vi "RemoteControl.TestLauncher.ConnectionMonitor.vi"(8 "error in (no error)":errorcluster, 11 "RC COM Type":T3=enum."ZMQ") -> (0 "error out":errorcluster)   [LabVIEW 2019, in "RemoteControl.lvclass"]
uses:
  RemoteControl.lvclass
  <vilib>/JKI/JKI SMO/SMO/Typedefs/SMOState --Enum.ctl
  Typedefs/PrivateEvents--RemoteControl.Configure.ctl
  Typedefs/RC Com Type--enum.ctl
  Typedefs/Message--Cluster.ctl
  Typedefs/RC Process Type--Enum.ctl
  RemoteControl.lvclass/RemoteControl.ctl
  <vilib>/JKI/JKI SMO/SMO/SMO.lvclass/SMO.ctl
  Typedefs/PrivateEvents--RemoteControl.SendMessageToProcess.ctl
  <vilib>/JKI/JKI SMO/SMO/Private/ReftoDVR--SMO.vi
  C:/Program Files (x86)/National Instruments/LabVIEW 2019/vi.lib/JKI/JKI SMO/SMO/SMO.lvclass
  <vilib>/JKI/JKI SMO/SMO/SMO.lvclass
panel:
  out "Response":T1={"Command"="Command3", "Data"=variant(string "Command: Command3\nTime: 10:01:32 AM\nGUID: 48148DED-56D8-49E7-9F94-E56068A2CC24"), "ID"="bc5bb9c457fa8484a73b80f0f0e9ae33"}
  in  "RC Process Type":T2=enum."Server"
  in  "Debug Mode":bool
  in  "Check Timing Mode":bool
  out "processed":i32=160
  out "Message":T1={"Command"="Command3", "Data"=variant(string[] ["[1433526]"]), "ID"="bc5bb9c457fa8484a73b80f0f0e9ae33"}
  in  "Configure":T4={"address"="*", "Port"=6341, "AllowedRemote"="", "Commands"=["Command1", "Command2", "Command3", "ACK", "HELP"], "timeout"=0}
  out "SMO State":T5=enum."Stopped"
  in  "Stop":bool
  # "RC SMO Test Launcher"
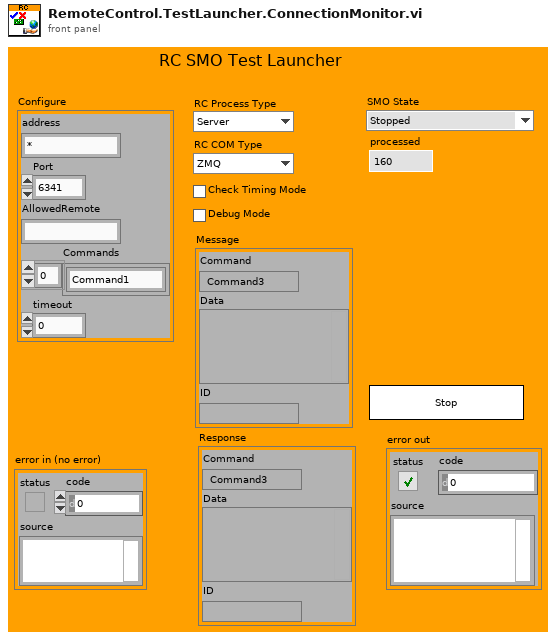
[diagram p1: front panel]
types:
  T1 = typedef "RemoteControl.lvclass/Message--Cluster.ctl" = cluster{"Command":string, "Data":variant, "ID":string}
  T2 = typedef "RemoteControl.lvclass/RC Process Type--Enum.ctl" = enum16{"Listener", "Server", "Client"}
  T3 = typedef "RemoteControl.lvclass/RC Com Type--enum.ctl" = enum16{"RC", "STM", "ZMQ"}
  T4 = typedef "RemoteControl.lvclass/PrivateEvents--RemoteControl.Configure.ctl" = cluster{"address":string, "Port":u16, "AllowedRemote":string, "Commands":string[], "timeout":i32}
  T5 = typedef "SMO.lvclass/SMOState --Enum.ctl" = enum16{"unknown", "Created", "Started", "Stopped"}
  T6 = typedef "SMO.lvclass/Public Events.ctl" = cluster{"Error":refnum<user-event>, "State":refnum<user-event>, "Reserve State":refnum<user-event>}
  T7 = typedef "RemoteControl.lvclass/PublicEvents--Cluster.ctl" = cluster{"SendMessageFromProcess":refnum<user-event>}
  T8 = typedef "RemoteControl.lvclass/PrivateEvents--RemoteControl.SendMessageToProcess.ctl" = cluster{"Message":T1}
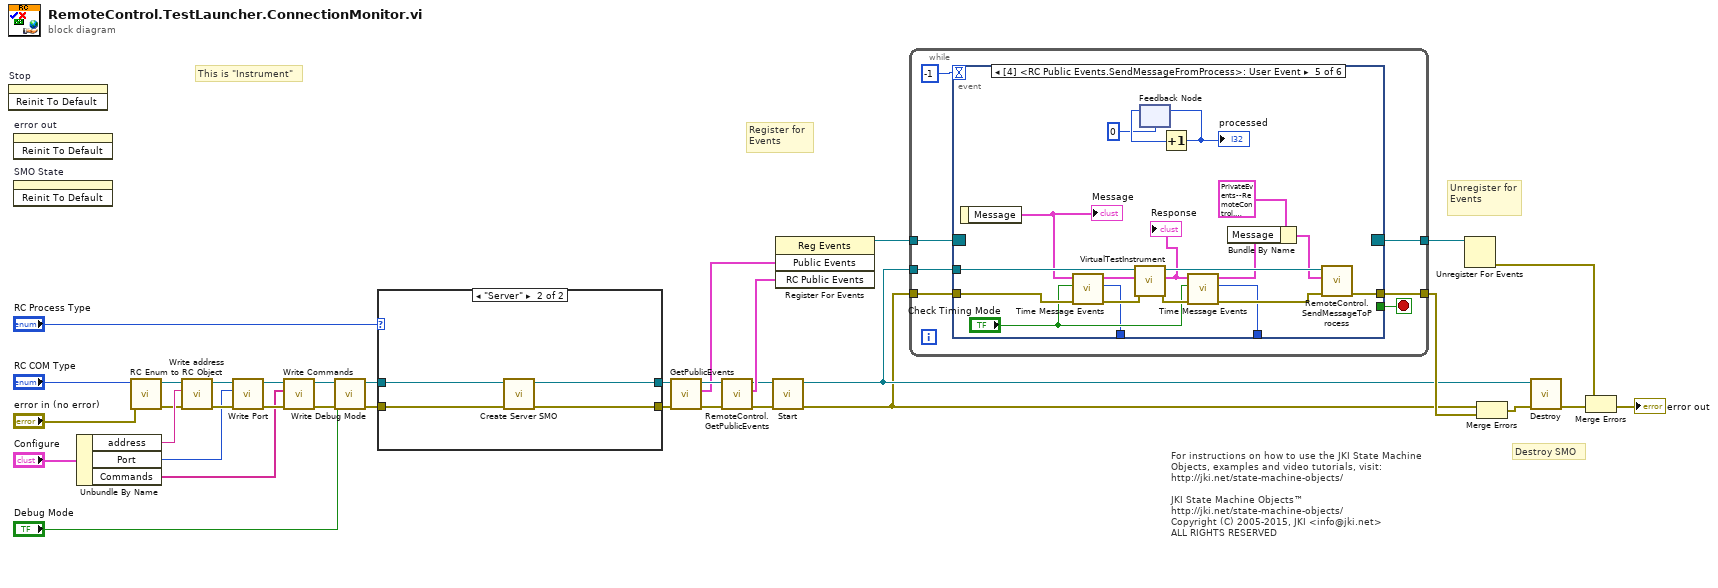
[diagram p0: block diagram]
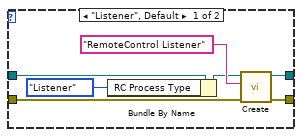
[diagram p2: hidden frame]
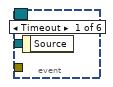
[diagram p3: hidden frame]
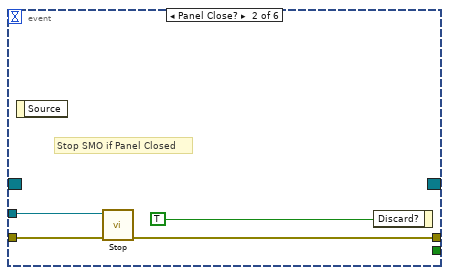
[diagram p4: hidden frame]
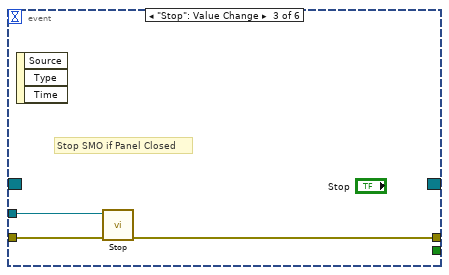
[diagram p5: hidden frame]
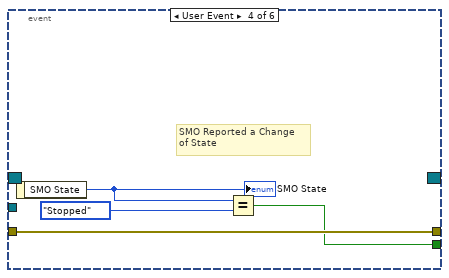
[diagram p6: hidden frame]
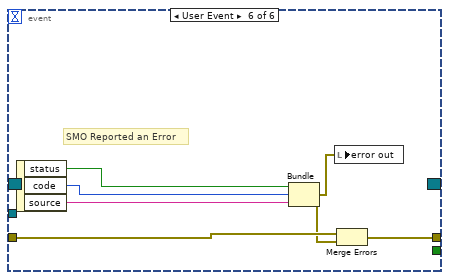
[diagram p7: hidden frame]
diagram:
  # "Register for Events"
  # "This is \"Instrument\""
  # "For instructions on how to use the JKI State Machine Objects, examples and video tutorials, visit:\nhttp://jki.net/state-machine-objects/\n\nJKI State Machine Objects™\nhttp://jki.net/state-machine-objects/\nCopyright (C) 2005-2015, JKI <info@jki.net>\nALL RIGHTS RESERVED"
  # "Destroy SMO"
  # "Unregister for Events"
  n1 = invoke on="Stop" class="Bool" method="Reinit To Default"() -> ()  [unwired: 3 in, 3 out]
  n2 = invoke on="error out" class="Clust (strict)" method="Reinit To Default"() -> ()  [unwired: 3 in, 3 out]
  n3 = invoke on="SMO State" class="Enum (strict)" method="Reinit To Default"() -> ()  [unwired: 3 in, 3 out]
  n4 = Unbundle By Name("Configure") -> ("address"=w6:string, "Port"=w5:u16, "Commands"=w4:string[])
  n5 = call "RC Enum to RC Object.vi"("error in (no error)"="error in (no error)", "RC Type"="RC COM Type") -> ("error out"=w1:errorcluster, "RemoteControl out"=w15:refnum<class "RemoteControl.lvclass">)  [unwired: 8 in]
  n6 = call-dynamic "Write address.vi"("error in (no error)"=w1, "address"=w6, "RemoteControl in"=w15) -> ("error out"=w22:errorcluster, "RemoteControl out"=w23:refnum<class "RemoteControl.lvclass">)  [unwired: 7 in]
  n7 = call-dynamic "Write Port.vi"("error in (no error)"=w22, "Port"=w5, "RemoteControl in"=w23) -> ("error out"=w20:errorcluster, "RemoteControl out"=w21:refnum<class "RemoteControl.lvclass">)  [unwired: 7 in]
  n8 = call-dynamic "Write Commands.vi"("error in (no error)"=w20, "Commands"=w4, "RemoteControl in"=w21) -> ("error out"=w19:errorcluster, "RemoteControl out"=w18:refnum<class "RemoteControl.lvclass">)  [unwired: 7 in]
  n9 = call "Write Debug Mode.vi"("error in (no error)"=w19, "Debug Mode?"="Debug Mode", "RemoteControl in"=w18) -> ("error out"=w7:errorcluster, "RemoteControl out"=w8:refnum<class "RemoteControl.lvclass">)  [unwired: 7 in]
  n10 = case shown="\"Server\"" "RC Process Type" {
    tunnel: [w39 w46] -> w14
    tunnel: [w40 w45] -> w13
    tunnel: w8 -> [w38 w44]
    tunnel: w7 -> [w37 w43]
    frame "Listener", Default {
      n11 = Bundle By Name(cluster=w38, "RC Process Type"=RC_Process_Type--Enum."Listener") -> (w36:refnum<class "RemoteControl.lvclass">)
      n12 = call <vilib>:"Create.vi"("error in (no error)"=w37, "Subsystem Name (optional)"="RemoteControl Listener" ("format string"), "SMO"=w36) -> ("error out"=w40:errorcluster, "SMO out"=w39:refnum<class "RemoteControl.lvclass">)  [unwired: 6 in, 1 out]
    }
    frame "Server" {
      n13 = call-dynamic "Create Server SMO.vi"("error in (no error)"=w43, "RemoteControl in"=w44) -> ("error out"=w45:errorcluster, "RemoteControl out"=w46:refnum<class "RemoteControl.lvclass">)  [unwired: 8 in]
    }
  }
  n14 = call <vilib>:"GetPublicEvents.vi"("error in (no error)"=w13, "SMO"=w14) -> ("error out"=w29:errorcluster, "Public Events"=w28:T6, "SMO out"=w30:refnum<class "RemoteControl.lvclass">)  [unwired: 7 in]
  n15 = call "RemoteControl.GetPublicEvents.vi"("error in (no error)"=w29, "RemoteControl"=w30) -> ("error out"=w12:errorcluster, "RC Public Events"=w26:T7, "RemoteControl out"=w11:refnum<class "RemoteControl.lvclass">)  [unwired: 7 in]
  n16 = call <vilib>:"Start.vi"("error in (no error)"=w12, "SMO"=w11) -> ("error out"=w9:errorcluster, "SMO out"=w10:refnum<class "RemoteControl.lvclass">)  [unwired: 8 in]
  n17 = register-events(w28, w26) -> (reference out=w27:refnum<event-registration>)  [unwired: 2 in, 1 out]
  n18 = while {
    tunnel: w27 -> [w50]
    tunnel: [w49] -> w35
    tunnel: w10 -> [w48]
    tunnel: w9 -> [w51]
    tunnel: [w52] -> w34
    stop <- w53 stop-if-true
    n19 = event shown="[4] <RC Public Events.SendMessageFromProcess>: User Event" {
      selector: w50 -> [_ _ _ _ _ _]
      dyn-events: [_ _ _ _ _ _] -> w49
      timeout: -1 -> [_ _ _ _ _ _]
      tunnel: [_ _ _ w61 _ _] -> w53
      tunnel: w48 -> [_ w57 w60 _ w78 _]
      tunnel: [_ w56 w59 w64 _ w87] -> w52
      tunnel: w51 -> [_ w55 w58 w64 w75 w85]
      tunnel: [_ _ _ _ w83 _] -> _
      tunnel: [_ _ _ _ w68 _] -> _
      tunnel: [_ _ _ _ w67 _] -> _
      event Timeout {
        n20 = event-data() -> ()  [unwired: 1 in, 1 out]
      }
      event Panel Close? {
        # "Stop SMO if Panel Closed"
        n21 = event-data() -> ()  [unwired: 1 in, 1 out]
        n22 = call <vilib>:"Stop.vi"("error in (no error)"=w55, "SMO"=w57) -> ("error out"=w56:errorcluster)  [unwired: 8 in, 1 out]
        n23 = event-data("Discard?"=TRUE ("OK")) -> ()  [unwired: 1 in, 1 out]
      }
      event "Stop": Value Change {
        # "Stop SMO if Panel Closed"
        n24 = event-data() -> ()  [unwired: 1 in, 3 out]
        n25 = call <vilib>:"Stop.vi"("error in (no error)"=w58, "SMO"=w60) -> ("error out"=w59:errorcluster)  [unwired: 8 in, 1 out]
      }
      event User Event {
        # "SMO Reported a Change\nof State"
        n26 = event-data() -> ("SMO State"=w63:T5)  [unwired: 1 in]
        "SMO State" <- w63
        n27 = Equal?(x=w63, y=SMOState_--Enum."Stopped") -> (x = y?=w61:bool)
      }
      event User Event {
        n28 = event-data() -> ("Message"=w76:T1)  [unwired: 1 in]
        "Message" <- w76
        n29 = call "Time Message Events.vi"("error in (no error)"=w75, "Debug Mode"="Check Timing Mode", "Message in"=w76) -> ("error out"=w74:errorcluster, "time (ms)"=w68:u32, "Message out"=w66:T1)  [unwired: 6 in]
        n30 = call "VirtualTestInstrument.vi"("error in (no error)"=w74, "Message"=w66, "RemoteControl"=w78) -> ("error out"=w71:errorcluster, "processed Message"=w65:T1, "RemoteControl"=w77:refnum<class "RemoteControl.lvclass">)  [unwired: 6 in]
        "Response" <- w65
        n31 = feedback #1(0) -> (w80:i32)
        n32 = Increment(x=w80) -> (x+1=w81:i32)
        "processed" <- w81
        n33 = feedback-in #1(w81) -> ()
        n34 = call "Time Message Events.vi"("error in (no error)"=w71, "Debug Mode"="Check Timing Mode", "Message in"=w65) -> ("error out"=w73:errorcluster, "time (ms)"=w67:u32, "Message out"=w70:T1)  [unwired: 6 in]
        n35 = Bundle By Name(cluster=T8 {"Message"={"Command"="", "Data"=variant(bool FALSE), "ID"=""}} ("SendMessgaeToProcess"), "Message"=w70) -> (w72:T8)
        n36 = call "RemoteControl.SendMessageToProcess.vi"("error in (no error)"=w73, "SendMessageToProcess"=w72, "RemoteControl"=w77) -> ("error out"=w83:errorcluster)  [unwired: 7 in, 1 out]
      }
      event User Event {
        # "SMO Reported an Error"
        n37 = event-data() -> ("status"=w86:bool, "code"=w89:i32, "source"=w88:string)  [unwired: 1 in]
        n38 = Bundle("status"=w86, "code"=w89, "source"=w88) -> (w84:errorcluster)  [unwired: 1 in]
        n39 = local write "error out"(w84) -> ()
        n40 = Merge Errors(w85, w84) -> (w87:errorcluster)
      }
    }
  }
  n41 = Unregister For Events(event registration refnum=w35) -> (error out=w33:errorcluster)  [unwired: 1 in]
  n42 = Merge Errors(w9, w34) -> (w25:errorcluster)
  n43 = call <vilib>:"Destroy.vi"("error in (no error)"=w25, "SMO"=w10) -> ("error out"=w31:errorcluster)  [unwired: 9 in]
  n44 = Merge Errors(w33, w31) -> (→"error out":errorcluster)
